vi "PWM Arduino.vi"() -> ()   [LabVIEW 2014]
uses:
  <vilib>/LabVIEW Interface for Arduino/Type Defs/Pin Mode.ctl
  <vilib>/LabVIEW Interface for Arduino/LabVIEW Interface for Arduino.lvlib
panel:
  in  "VISA resource name":refnum<visa-resource-name>
  in  "Horizontal Pointer Slide":dbl(slide) scale=0.0..100.0
  # "Arduino COM Select"
  # "Duty Cycle Adjust [%]"
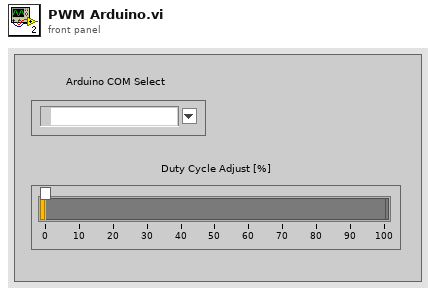
[diagram p1: front panel]
types:
  T1 = typedef "LabVIEW Interface for Arduino.lvlib/Pin Mode.ctl" = enum8{"Input", "Output"}
  T2 = typedef "LabVIEW Interface for Arduino.lvlib/Arduino Resource.ctl" = cluster{"VISA resource":refnum<visa-resource-name>, "Board Type":T3, "Connection Type":enum8{"USB / Serial"}, "Bytes Per Packet (15)":u8}
  T3 = typedef "LabVIEW Interface for Arduino.lvlib/Board Type.ctl" = enum16{"Uno", "Dimuelanove w/Atmega 328", "Mega 2560"}
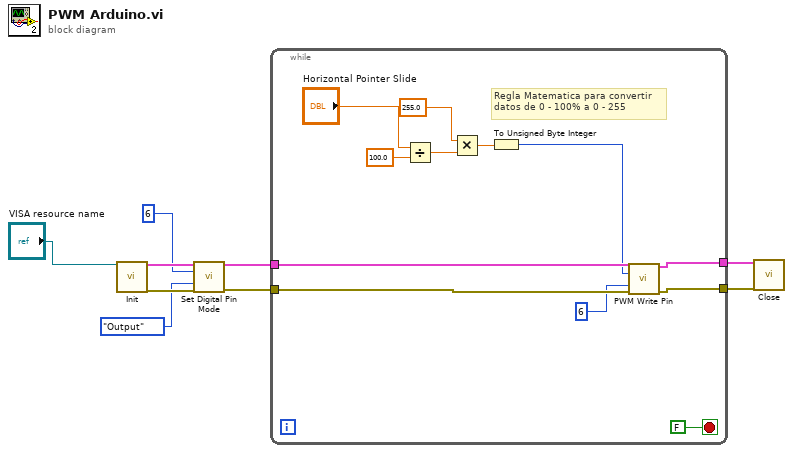
[diagram p0: block diagram]
diagram:
  n1 = call <vilib>:"Init.vi"("VISA resource"="VISA resource name") -> ("Arduino Resource"=w6:T2, "error out"=w9:errorcluster)  [unwired: 17 in]
  n2 = call <vilib>:"Set Digital Pin Mode.vi"("Arduino Resource"=w6, "Digital I/O Pin"=u8 6, "Pin Mode (Input)"=Pin_Mode."Output", "error in"=w9) -> ("Arduino Resource"=w5:T2, "error out"=w8:errorcluster)  [unwired: 10 in]
  n3 = while {
    tunnel: w8 -> [w21]
    tunnel: [w20] -> w7
    tunnel: w5 -> [w19]
    tunnel: [w18] -> w4
    stop <- FALSE stop-if-true
    # "Regla Matematica para convertir\ndatos de 0 - 100% a 0 - 255"
    n4 = Divide(x="Horizontal Pointer Slide", y=100.0) -> (x/y=w15:dbl)
    n5 = Multiply(x=255.0, y=w15) -> (x*y=w13:dbl)
    n6 = To Unsigned Byte Integer(number=w13) -> (unsigned 8bit integer=w12:u8)
    n7 = call <vilib>:"PWM Write Pin.vi"("Arduino Resource"=w19, "Duty Cycle (0 - 255)"=w12, "PWM Pin (3)"=u8 6, "error in"=w21) -> ("Arduino Resource"=w18:T2, "error out"=w20:errorcluster)  [unwired: 10 in]
  }
  n8 = call <vilib>:"Close.vi"("Arduino Resource"=w4, "error in"=w7) -> ()  [unwired: 13 in, 1 out]
